vi "SoftTriggerEnable.vi"() -> ()   [LabVIEW 2017]
panel:
  in  "address":string="192.168.10.20"
  out "error out":errorcluster
  in  "SoftTriggerEnable":bool=TRUE
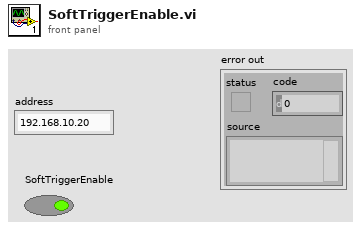
[diagram p1: front panel]
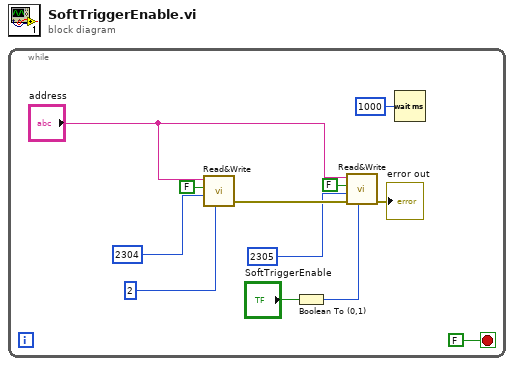
[diagram p0: block diagram]
diagram:
  n1 = while {
    stop <- FALSE stop-if-true
    n2 = call "Read&Write.vi"("In"=u8 2, "Address"=u32 2304, "Read (TRUE)"=FALSE, "address"="address") -> ("error out"=w11:errorcluster)  [unwired: 6 in, 1 out]
    n3 = Boolean To (0,1)(Boolean="SoftTriggerEnable") -> (0, 1=w5:i16)
    n4 = call "Read&Write.vi"("In"=w5, "error in (no error)"=w11, "Address"=u32 2305, "Read (TRUE)"=FALSE, "address"="address") -> ("error out"=→"error out":errorcluster)  [unwired: 5 in, 1 out]
    n5 = Wait (ms)(milliseconds to wait=u32 1000) -> ()  [unwired: 1 out]
  }
